vi "FileIO-Write Parameters.vi"(0 "Parameter File":path, 2 "Default Folder":path, 5 "Parameters":variant, 9 "Prompt? (T)":bool=TRUE, 11 "error in (no error)":errorcluster) -> (4 "selected path":path, 8 "saved":bool, 15 "error out":errorcluster)   [LabVIEW 2020]
panel:
  out "Version":i32
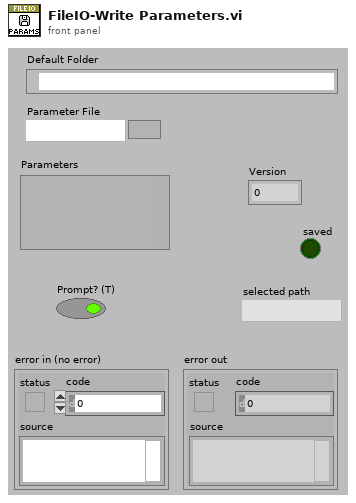
[diagram p1: front panel]
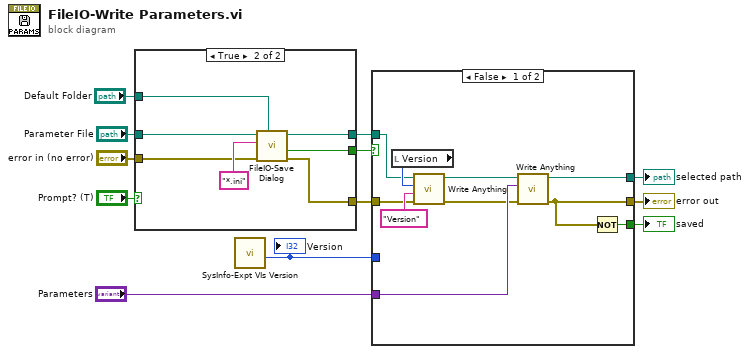
[diagram p0: block diagram]
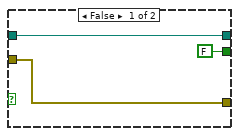
[diagram p2: hidden frame]
diagram:
  n1 = case shown="True" "Prompt? (T)" {
    tunnel: [FALSE ("cancelled") w22] -> w10
    tunnel: [w14 w21] -> w9
    tunnel: [w13 w20] -> w6
    tunnel: "Parameter File" -> [w14 w18]
    tunnel: "error in (no error)" -> [w13 w17]
    tunnel: "Default Folder" -> [_ w16]
    frame False {
    }
    frame True {
      n2 = call "FileIO-Save Dialog.vi"("Default Folder"=w16, "error in"=w17, "pattern (all files)"="*.ini", "Start path"=w18) -> ("error out"=w20:errorcluster, "cancelled"=w22:bool, "selected path"=w21:path)  [unwired: 5 in]
    }
  }
  n3 = call "SysInfo-Expt VIs Version.vi"() -> ("Expt VIs Version out"=w5:i32)  [unwired: 11 in]
  "Version" <- w5
  n4 = case shown="False" w10 {
    tunnel: [w23 w34] -> w12
    tunnel: "Parameters" -> [w32 _]
    tunnel: w9 -> [w29 w33]
    tunnel: w6 -> [w28 w34]
    tunnel: w5 -> [_ _]
    tunnel: [w27 _] -> w4
    tunnel: [w24 w33] -> w3
    frame False {
      n5 = local read "Version"() -> (w31:i32)
      n6 = call "Write Anything.vi"("Error In"=w28, "Section Name (Name of \"Anything\")"="Version" ("Section Name (Name of \"Anything\")"), "Anything"=w31, "Path (dialog)"=w29) -> ("Error Out"=w26:errorcluster, "Path out"=w25:path)  [unwired: 6 in]
      n7 = call "Write Anything.vi"("Error In"=w26, "Anything"=w32, "Path (dialog)"=w25) -> ("Error Out"=w23:errorcluster, "Path out"=w24:path)  [unwired: 7 in]
      n8 = Not(x=w23) -> (.not. x?=w27:bool)
    }
    frame True {
    }
  }
  "error out" <- w12
  "saved" <- w4
  "selected path" <- w3
